vi "RW Annlus ROI.vi"(7 "Read/Write":enum16{"Read", "Write"}(ring), 8 "error in (no error)":errorcluster, 9 "directory Path":string="Ini\\ROI.ini", 10 "section":string, 11 "ROI Descriptor":T1 {"Contours"."Type" items=["No Selection", "Point", "Line", "Rectangle", "Oval", "Polygon", "Freehand Region", "Annulus", "Unused2", "Unused3", "Broken Line", "Freehand Line", "Rotated Rectangle"]}) -> (0 "error out":errorcluster, 3 "ROI Descriptor Out":T1 {"Contours"."Type" items=["No Selection", "Point", "Line", "Rectangle", "Oval", "Polygon", "Freehand Region", "Annulus", "Unused2", "Unused3", "Broken Line", "Freehand Line", "Rotated Rectangle"]})   [LabVIEW 2017]
uses:
  File/Control/Parent path.ctl
  <vilib>/Utility/config.llb/Write Key (I32).vi
  <vilib>/Utility/config.llb/Write Key (Double).vi
  <vilib>/Utility/config.llb/Read Key (I32).vi
  <vilib>/Utility/config.llb/Read Key (Double).vi
  File/File.lvlib
  <vilib>/Utility/config.llb/NI_LVConfig.lvlib
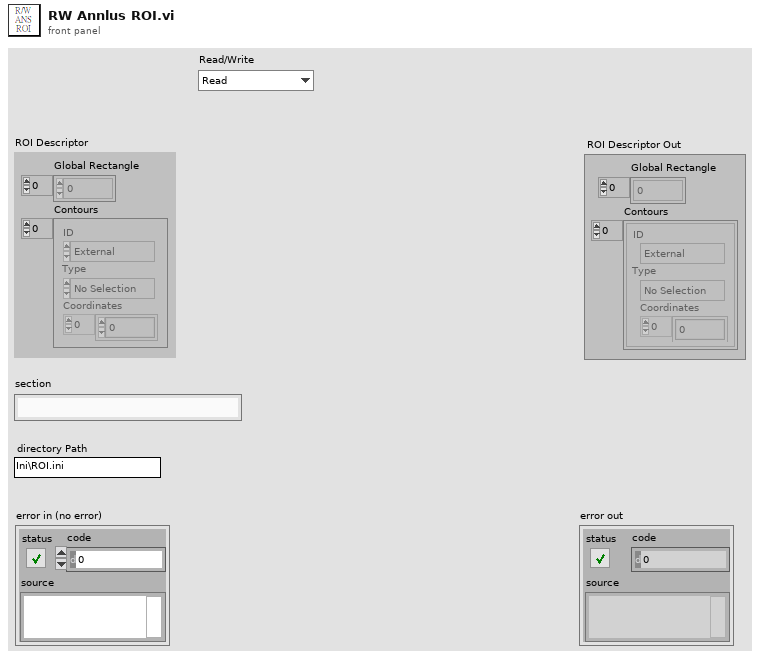
[diagram p1: front panel]
types:
  T1 = typedef "ROI Descriptor" = cluster{"Global Rectangle":i32[], "Contours":cluster{"ID":enum32{"External", "Internal"}, "Type":u32, "Coordinates":i32[]}[]}
  T2 = typedef "File.lvlib/Parent path.ctl" = enum16{"Project", "Setting", "Log"}
  T3 = typedef "NI_LVConfig.lvlib/Config Data RefNum.ctl" = refnum<k1>
  T4 = typedef "IMAQ Circle" = cluster{"Center X":i32, "Center Y":i32, "Inner Radius":i32, "Outer Radius":i32, "Start Angle":dbl, "End Angle":dbl}
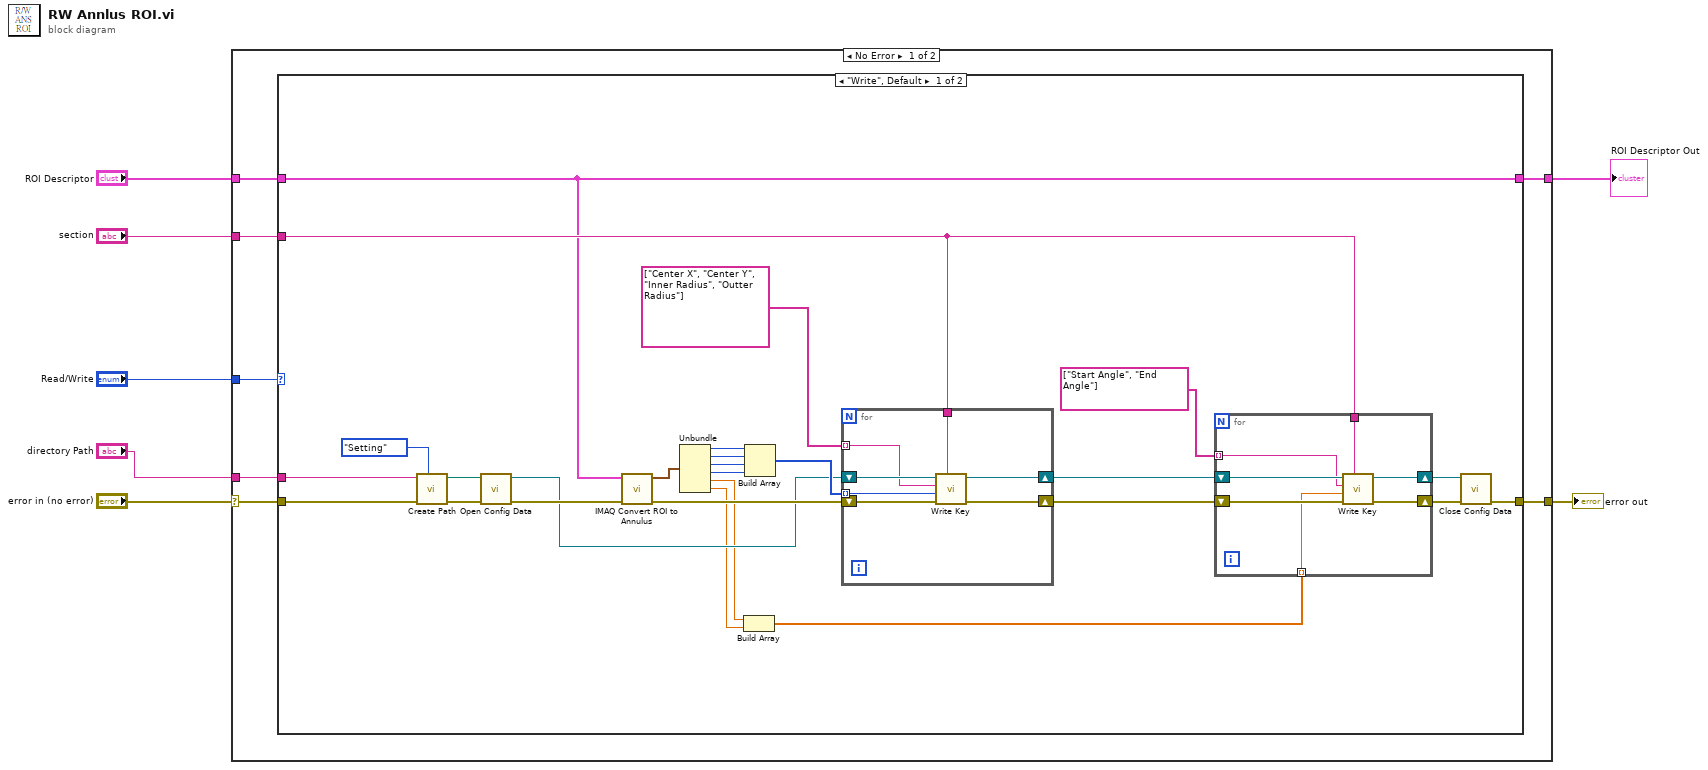
[diagram p0: block diagram]
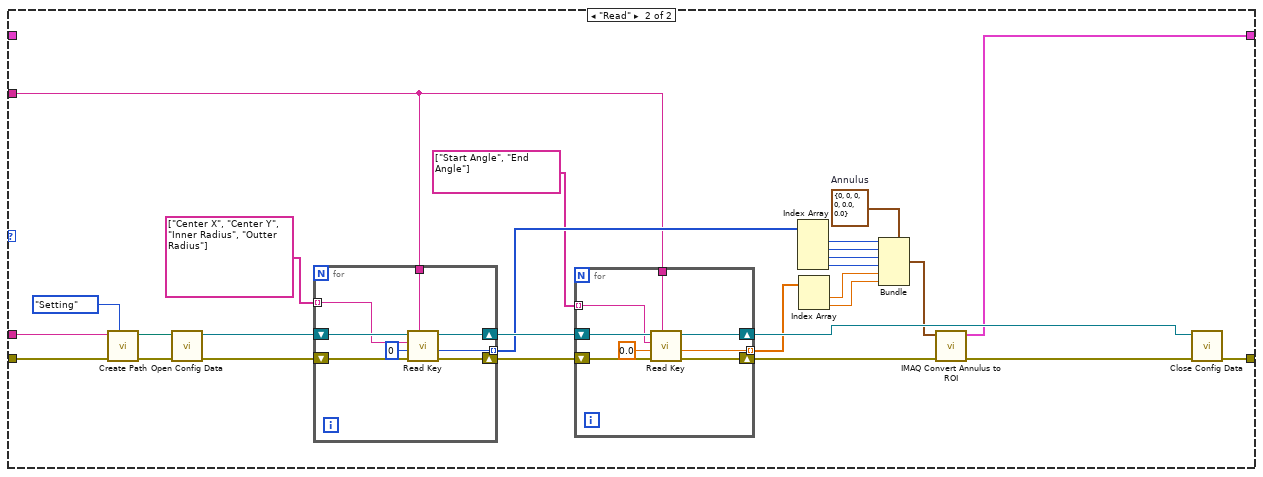
[diagram p2: hidden frame]
diagram:
  n1 = case shown="No Error" "error in (no error)" {
    selector: "error in (no error)" -> [w14 w99]
    tunnel: [w13 w99] -> w6
    tunnel: "Read/Write" -> [w12 _]
    tunnel: "section" -> [w11 _]
    tunnel: "directory Path" -> [w10 _]
    tunnel: "ROI Descriptor" -> [w9 w98]
    tunnel: [w8 w98] -> w1
    frame No Error {
      n2 = case shown="\"Write\", Default" w12 {
        tunnel: w14 -> [w40 w81]
        tunnel: [w34 w75] -> w13
        tunnel: w11 -> [w22 w64]
        tunnel: w10 -> [w21 w60]
        tunnel: w9 -> [w20 _]
        tunnel: [w20 w61] -> w8
        frame "Write", Default {
          n3 = call "Create Path.vi"("Parent path"=Parent_path."Setting", "error in (no error)"=w40, "Directory"=w21) -> ("error out"=w38:errorcluster, "Path"=w37:path)  [unwired: 7 in]
          n4 = call <vilib>:"Open Config Data.vi"("error in (no error)"=w38, "configuration file path"=w37) -> ("error out"=w36:errorcluster, "refnum"=w23:T3)  [unwired: 7 in, 1 out]
          n5 = call "IMAQ Convert ROI to Annulus"("error in (no error)"=w36, "ROI Descriptor"=w20) -> ("error out"=w30:errorcluster, "Annulus"=w29:T4)  [unwired: 7 in]
          n6 = Unbundle(w29) -> ("Center X"=w28:i32, "Center Y"=w27:i32, "Inner Radius"=w26:i32, "Outer Radius"=w25:i32, "Start Angle"=w19:dbl, "End Angle"=w18:dbl)
          n7 = Build Array(w19, w18) -> (w17:dbl[])
          n8 = Build Array(w28, w27, w26, w25) -> (w24:i32[])
          n9 = for {
            shift-right: [w52] -> w32
            shift-left: w23 -> [w54]
            shift-right: [w51] -> w31
            shift-left: w30 -> [w53]
            tunnel: string[] ["Center X", "Center Y", "Inner Radius", "Outter Radius"] ("Rect") -> [w50] mode=indexing
            tunnel: w22 -> [w49]
            tunnel: w24 -> [w48] mode=indexing
            n10 = call-poly <vilib>:"Write Key.vi"("section"=w49, "error in (no error)"=w53, "value"=w48, "key"=w50, "refnum"=w54) -> ("error out"=w51:errorcluster, "refnum out"=w52:T3)  [unwired: 4 in, 1 out]
          }
          n11 = for {
            tunnel: w22 -> [w43]
            shift-right: [w46] -> w33
            shift-left: w32 -> [w45]
            shift-right: [w47] -> w35
            shift-left: w31 -> [w44]
            tunnel: w17 -> [w42] mode=indexing
            tunnel: string[] ["Start Angle", "End Angle"] ("Rect") -> [w41] mode=indexing
            n12 = call-poly <vilib>:"Write Key.vi"("section"=w43, "error in (no error)"=w44, "value"=w42, "key"=w41, "refnum"=w45) -> ("error out"=w47:errorcluster, "refnum out"=w46:T3)  [unwired: 4 in, 1 out]
          }
          n13 = call <vilib>:"Close Config Data.vi"("error in (no error)"=w35, "refnum"=w33) -> ("error out"=w34:errorcluster)  [unwired: 8 in, 1 out]
        }
        frame "Read" {
          w58 = T4 {"Center X"=0, "Center Y"=0, "Inner Radius"=0, "Outer Radius"=0, "Start Angle"=0.0, "End Angle"=0.0}  # Annulus
          n14 = call "Create Path.vi"("Parent path"=Parent_path."Setting", "error in (no error)"=w81, "Directory"=w60) -> ("error out"=w79:errorcluster, "Path"=w78:path)  [unwired: 7 in]
          n15 = call <vilib>:"Open Config Data.vi"("error in (no error)"=w79, "configuration file path"=w78) -> ("error out"=w76:errorcluster, "refnum"=w77:T3)  [unwired: 7 in, 1 out]
          n16 = for {
            shift-right: [w95] -> w73
            shift-left: w77 -> [w97]
            shift-right: [w94] -> w72
            shift-left: w76 -> [w96]
            tunnel: [w93] -> w70 mode=indexing
            tunnel: string[] ["Center X", "Center Y", "Inner Radius", "Outter Radius"] ("Rect") -> [w92] mode=indexing
            tunnel: w64 -> [w91]
            n17 = call-poly <vilib>:"Read Key.vi"("section"=w91, "error in (no error)"=w96, "default value"=0, "key"=w92, "refnum"=w97) -> ("error out"=w94:errorcluster, "value"=w93:i32, "refnum out"=w95:T3)  [unwired: 3 in, 1 out]
          }
          n18 = for {
            tunnel: [w85] -> w65 mode=indexing
            tunnel: w64 -> [w83]
            shift-right: [w89] -> w74
            shift-left: w73 -> [w88]
            shift-right: [w86] -> w71
            shift-left: w72 -> [w87]
            tunnel: string[] ["Start Angle", "End Angle"] ("Rect") -> [w82] mode=indexing
            n19 = call-poly <vilib>:"Read Key.vi"("section"=w83, "error in (no error)"=w87, "default value"=0.0, "key"=w82, "refnum"=w88) -> ("error out"=w86:errorcluster, "value"=w85:dbl, "refnum out"=w89:T3)  [unwired: 3 in, 1 out]
          }
          n20 = Index Array(array=w70) -> (element #1=w69:i32, element #2=w68:i32, element #3=w67:i32, element #4=w66:i32)  [unwired: 4 in]
          n21 = Index Array(array=w65) -> (element #1=w57:dbl, element #2=w56:dbl)  [unwired: 2 in]
          n22 = Bundle(cluster=w58, "Center X"=w69, "Center Y"=w68, "Inner Radius"=w67, "Outer Radius"=w66, "Start Angle"=w57, "End Angle"=w56) -> (w55:T4)
          n23 = call "IMAQ Convert Annulus to ROI"("error in (no error)"=w71, "Annulus"=w55) -> ("error out"=w62:errorcluster, "ROI Descriptor"=w61:T1)  [unwired: 7 in]
          n24 = call <vilib>:"Close Config Data.vi"("error in (no error)"=w62, "refnum"=w74) -> ("error out"=w75:errorcluster)  [unwired: 8 in, 1 out]
        }
      }
    }
    frame Error {
    }
  }
  "error out" <- w6
  "ROI Descriptor Out" <- w1
